vi "Send Command.vi"(0 "reference in":refnum<class "UE_master.lvclass">, 5 "message":string, 7 "parameters":string, 9 "data":variant, 11 "error in (no error)":errorcluster, 12 "response?":bool, 13 "timeout":i32=500) -> (4 "reference out":refnum<class "UE_master.lvclass">, 6 "status":string, 8 "reponse":string, 10 "data":variant, 15 "error out":errorcluster)   [LabVIEW 2019, in "CommandResponse communication.lvlib" / "UE_master.lvclass"]
doc: "Sends command as message + variant data and optionally awaits for response message and error"
uses:
  UE_master.lvclass
  Command + data + response cluster.ctl
  Status + response + data cluster.ctl
  CommandResponse communication.lvlib
  <vilib>/addons/_JKI.lib/Serialization/JSON/JKI JSON Serialization.lvlib
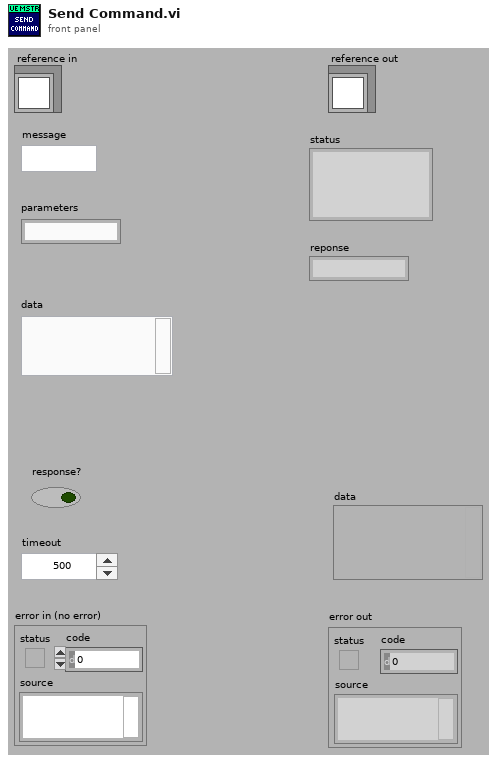
[diagram p1: front panel]
types:
  T1 = typedef "CommandResponse communication.lvlib/Status + response + data cluster.ctl" = cluster{"message":string, "response":string, "data":variant}
  T2 = typedef "CommandResponse communication.lvlib/Command + data + response cluster.ctl" = cluster{"message":string, "parameters":string, "response notifier":refnum<notifier>, "data":variant}
  T3 = typedef "CommandResponse communication.lvlib/UE_master.lvclass/ObjectAttributes.ctl" = cluster{"Command UE":refnum<user-event>}
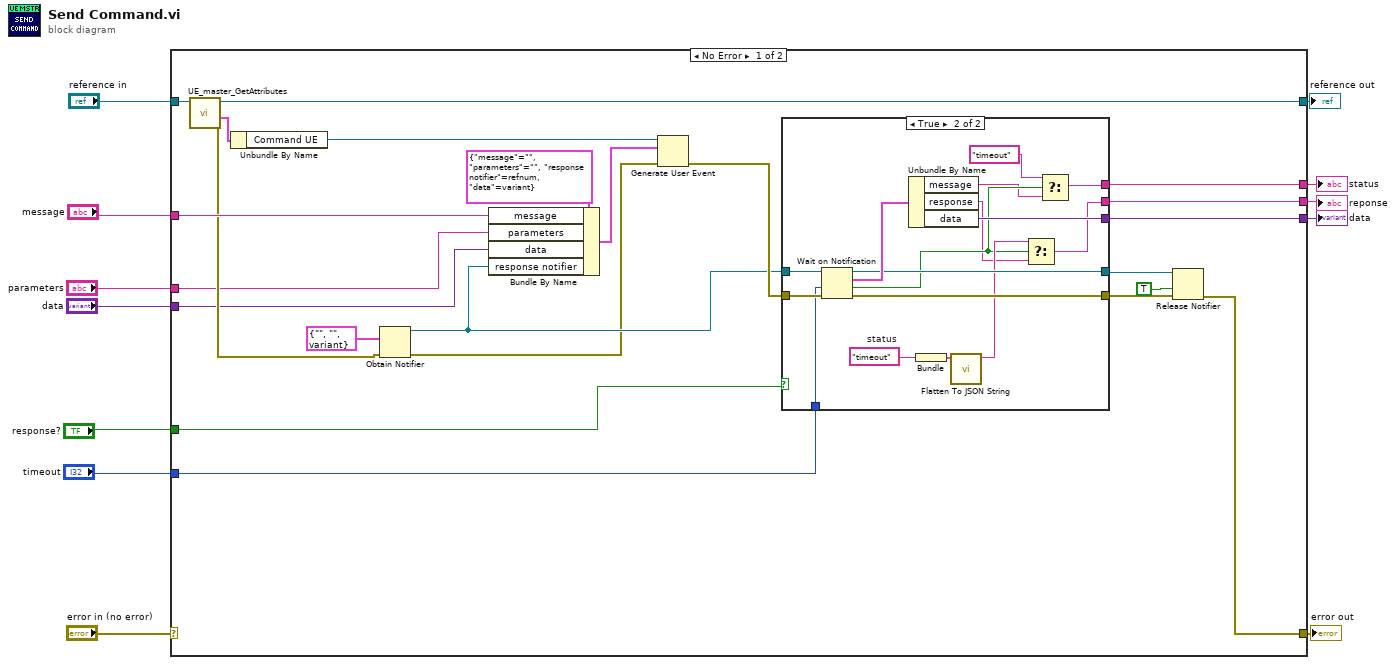
[diagram p0: block diagram]
diagram:
  n1 = case shown="No Error" "error in (no error)" {
    selector: "error in (no error)" -> [_ w55]
    tunnel: [w16 w55] -> w11
    tunnel: [w35 w54] -> w9
    tunnel: "reference in" -> [w33 w54]
    tunnel: "message" -> [w22 _]
    tunnel: "parameters" -> [w14 _]
    tunnel: "response?" -> [w21 _]
    tunnel: "timeout" -> [w20 _]
    tunnel: [w19 _] -> w4
    tunnel: [w18 _] -> w3
    tunnel: [w17 _] -> w2
    tunnel: "data" -> [w13 _]
    frame No Error {
      n2 = call "UE_master_GetAttributes.vi"("reference in"=w33) -> ("error out"=w15:errorcluster, "attributes"=w34:T3, "reference out"=w35:refnum<class "UE_master.lvclass">)  [unwired: 7 in, 1 out]
      n3 = Unbundle By Name(w34) -> ("Command UE"=w23:refnum<user-event>)
      n4 = Obtain Notifier(notification data type=T1 {"message"="", "response"="", "data"=variant} ("notification"), error in (no error)=w15) -> (notifier out=w29:refnum<notifier>, error out=w28:errorcluster)  [unwired: 2 in, 1 out]
      n5 = Bundle By Name(cluster=T2 {"message"="", "parameters"="", "response notifier"=refnum, "data"=variant} ("event data"), "message"=w22, "parameters"=w14, "data"=w13, "response notifier"=w29) -> (w27:T2)
      n6 = Generate User Event(user event=w23, event data cluster=w27, error in=w28) -> (error out=w32:errorcluster)  [unwired: 1 in, 1 out]
      n7 = case shown="True" w21 {
        tunnel: w32 -> [w36 w53]
        tunnel: w29 -> [w37 w51]
        tunnel: [w37 w50] -> w26
        tunnel: [w36 w49] -> w24
        tunnel: [_ w39] -> w19
        tunnel: [_ w46] -> w18
        tunnel: w20 -> [_ w48]
        tunnel: [_ w47] -> w17
        frame False {
        }
        frame True {
          w45 = "timeout"  # status
          n8 = Wait on Notification(notifier=w51, timeout in ms (-1)=w48, error in (no error)=w53) -> (notifier out=w50:refnum<notifier>, notification=w52:T1, timed out?=w42:bool, error out=w49:errorcluster)  [unwired: 1 in]
          n9 = Unbundle By Name(w52) -> ("message"=w40:string, "response"=w41:string, "data"=w47:variant)
          n10 = Bundle("status"=w45) -> (w44:cluster{"status":string})  [unwired: 1 in]
          n11 = call <vilib>:"Flatten To JSON String.vi"("Variant"=w44) -> ("JSON String"=w43:string)  [unwired: 9 in, 1 out]
          n12 = Select(t=w43, s=w42, f=w41) -> (s? t:f=w46:string)
          n13 = Select(t="timeout", s=w42, f=w40) -> (s? t:f=w39:string)
        }
      }
      n14 = Release Notifier(notifier=w26, force destroy? (F)=TRUE, error in (no error)=w24) -> (error out=w16:errorcluster)  [unwired: 2 out]
    }
    frame Error {
    }
  }
  "error out" <- w11
  "reference out" <- w9
  "status" <- w4
  "reponse" <- w3
  "data" <- w2
